vi "Get Classes to Inherit From.vi"(8 "error in (no error)":errorcluster, 11 "New Class Dialog In":refnum<class "New Class Dialog.lvclass">) -> (0 "error out":errorcluster, 3 "New Class Dialog Out":refnum<class "New Class Dialog.lvclass">)   [LabVIEW 2020, in "New Class Dialog.lvclass"]
uses:
  New Class Dialog.lvclass
  Framework/Process/Process.lvclass
panel:
  out "Array":string[](array[string])
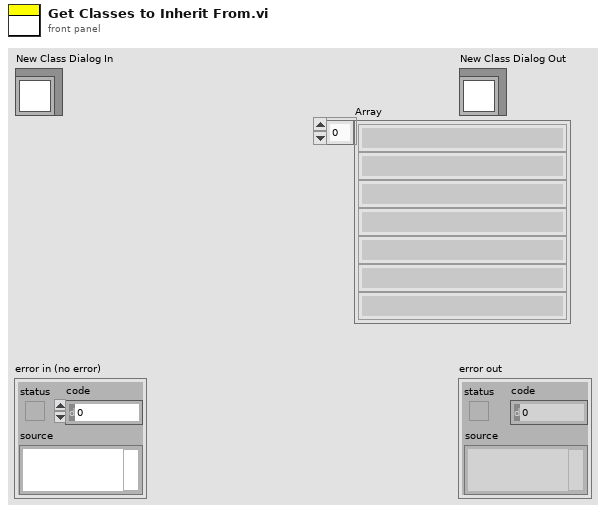
[diagram p1: front panel]
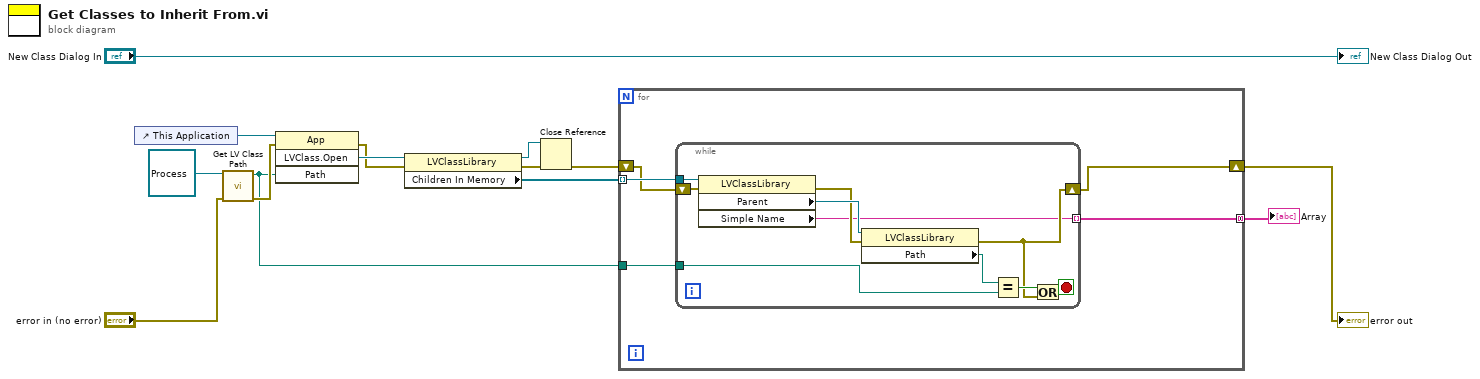
[diagram p0: block diagram]
diagram:
  n1 = control-ref of="This Application"() -> (w13:refnum<vi>)
  n2 = call <vilib>:"Get LV Class Path.vi"("error in (no error)"="error in (no error)", "object"=refnum<class "Process.lvclass"> refnum ("Process.lvclass")) -> ("error out"=w10:errorcluster, "class path"=w3:path)  [unwired: 8 in]
  n3 = invoke class="App" method="LVClass.Open"(reference=w13, error in=w10, "Path"=w3) -> (error out=w6:errorcluster, "LVClass.Open"=w9:refnum<vi>)  [unwired: 1 in, 2 out]
  n4 = property class="LVClassLibrary"(reference=w9, error in=w6) -> (reference out=w7:refnum<vi>, error out=w8:errorcluster, "Children In Memory"=w5:refnum<vi>[])
  n5 = Close Reference(reference=w7, error in (no error)=w8) -> (error out=w4:errorcluster)
  n6 = for {
    tunnel: w5 -> [w19] mode=indexing
    shift-right: [w16] -> w2
    shift-left: w4 -> [w17]
    tunnel: w3 -> [w18]
    tunnel: [w15] -> w1 mode=concatenating
    n7 = while {
      tunnel: w19 -> [w29]
      tunnel: w18 -> [w25]
      shift-right: [w22] -> w16
      shift-left: w17 -> [w24]
      tunnel: [w20] -> w15 mode=indexing
      stop <- w23 stop-if-true
      n8 = property class="LVClassLibrary"(reference=w29, error in=w24) -> (error out=w21:errorcluster, "Parent"=w28:refnum<vi>, "Simple Name"=w20:string)  [unwired: 1 out]
      n9 = property class="LVClassLibrary"(reference=w28, error in=w21) -> (error out=w22:errorcluster, "Path"=w27:path)  [unwired: 1 out]
      n10 = Equal?(x=w27, y=w25) -> (x = y?=w26:bool)
      n11 = Or(x=w26, y=w22) -> (x .or. y?=w23:bool)
    }
  }
  "error out" <- w2
  "Array" <- w1
  "New Class Dialog Out" <- "New Class Dialog In"
